vi "DDVL Reload VI.vi"(0 "Sub Panel Refs":refnum<vi>[](array[refnum]), 2 "Index":i32, 11 "Path/Ref Array In":T1(array[cluster])) -> (15 "Updated Path/Ref Array":T1(array[cluster]))   [LabVIEW 2016]
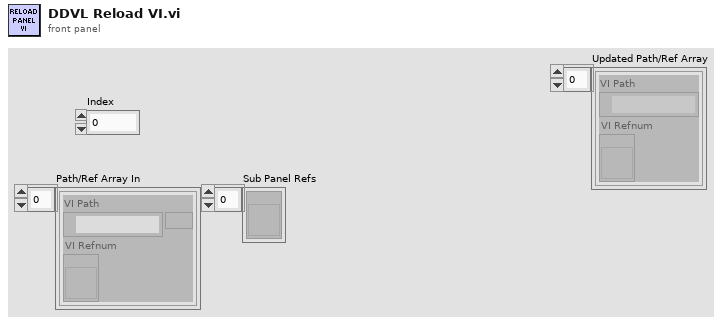
[diagram p1: front panel]
types:
  T1 = cluster{"VI Path":path, "VI Refnum":refnum<vi>}[]
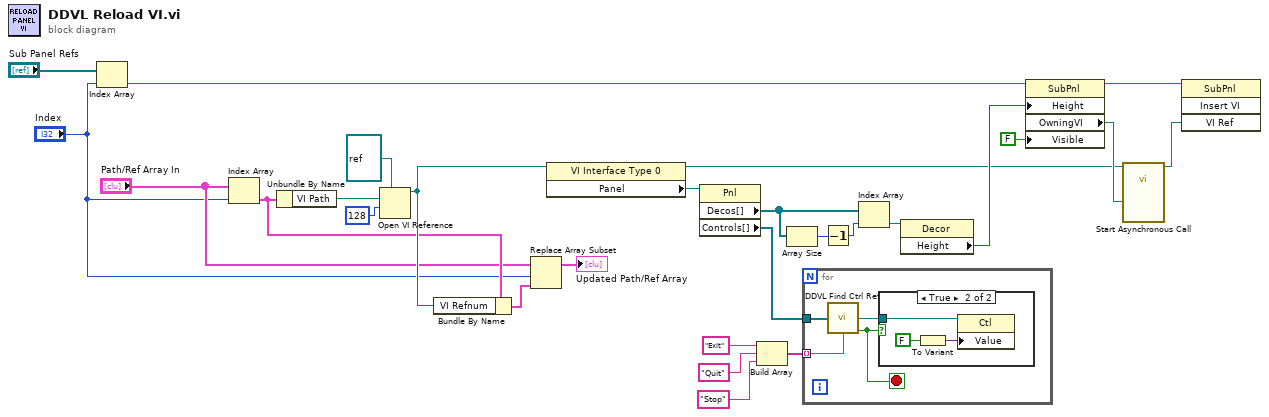
[diagram p0: block diagram]
diagram:
  n1 = Index Array(array="Sub Panel Refs", index="Index") -> (element=w21:refnum<vi>)
  n2 = Index Array(array="Path/Ref Array In", index="Index") -> (element=w15:cluster{"VI Path":path, "VI Refnum":refnum<vi>})
  n3 = Unbundle By Name(w15) -> ("VI Path"=w14:path)
  n4 = Open VI Reference(type specifier VI Refnum (for type only)=refnum<vi> refnum, vi path=w14, options=128) -> (vi reference=w17:refnum<vi>)  [unwired: 3 in, 1 out]
  n5 = Bundle By Name(cluster=w15, "VI Refnum"=w17) -> (w16:cluster{"VI Path":path, "VI Refnum":refnum<vi>})
  n6 = Replace Array Subset(array="Path/Ref Array In", new element=w16, index="Index") -> (→"Updated Path/Ref Array":T1)
  n7 = property class="VI Interface Type 0"(reference=w17) -> (reference out=w20:refnum<vi>, "Panel"=w23:refnum<vi>)  [unwired: 1 in, 1 out]
  n8 = property class="Pnl"(reference=w23) -> ("Decos[]"=w3:refnum<vi>[], "Controls[]"=w4:refnum<vi>[])  [unwired: 1 in, 2 out]
  n9 = Build Array("Exit" ("Control Label"), "Quit" ("Control Label"), "Stop" ("Control Label")) -> (w5:string[])
  n10 = Array Size(array=w3) -> (size(s)=w2:i32)
  n11 = for {
    tunnel: w4 -> [w31]
    tunnel: w5 -> [w29] mode=indexing
    stop <- w28 stop-if-true
    n12 = call "DDVL Find Ctrl Ref.vi"("Control Array"=w31, "Control Label"=w29) -> ("Control Ref"=w30:refnum<vi>, "Control Found?"=w28:bool)  [unwired: 12 in]
    n13 = case shown="True" w28 {
      tunnel: w30 -> [_ w34]
      frame False {
      }
      frame True {
        n14 = To Variant(anything=FALSE) -> (Variant=w33:variant)
        n15 = property class="Ctl"(reference=w34, "Value"=w33) -> ()  [unwired: 1 in, 2 out]
      }
    }
  }
  n16 = Decrement(x=w2) -> (x-1=w1:i32)
  n17 = Index Array(array=w3, index=w1) -> (element=w24:refnum<vi>)
  n18 = property class="Decor"(reference=w24) -> ("Height"=w25:u32)  [unwired: 1 in, 2 out]
  n19 = property class="SubPnl"(reference=w21, "Height"=w25, "Visible"=FALSE) -> (reference out=w22:refnum<vi>, "OwningVI"=w26:refnum<vi>)  [unwired: 1 in, 1 out]
  n20 = call-by-ref "Start Asynchronous Call"(reference=w20, "Calling VI Ref"=w26) -> (reference out=w9:refnum<vi>)  [unwired: 16 in, 1 out]
  n21 = invoke class="SubPnl" method="Insert VI"(reference=w22, "VI Ref"=w9) -> ()  [unwired: 2 in, 4 out]
